vi "measconfig parse section.vi"(8 "error in (no error)":errorcluster, 10 "section name":string, 11 "refnum":T1) -> (0 "error out":errorcluster, 2 "measurement definition":T2={"sweep parameter"=enum."angle", "sweep start"=0.0, "sweep stop"=0.0, "sweep increment"=0.0, "temperature"=0.0, "path"=path "", "magnet initial"={"magnitude"=0.0, "phi"=0.0, "theta"=0.0}, "magnet reference"={"magnitude"=0.0, "phi"=0.0, "theta"=0.0}, "const phi?"=FALSE, "delta phi (deg)"=0.5, "delta H (mT)"=0.5, "const phi init field?"=FALSE}, 3 "refnum out":T1)   [LabVIEW 2013]
uses:
  <vilib>/Utility/config.llb/Config Data RefNum.ctl
  measconfig cluster.ctl
  measurement sweep parameter.ctl
  devices/magnet/magnet polar field.ctl
  <vilib>/Utility/config.llb/Read Key (String).vi
  <vilib>/Utility/config.llb/Read Key (Double).vi
  <vilib>/Utility/config.llb/NI_LVConfig.lvlib
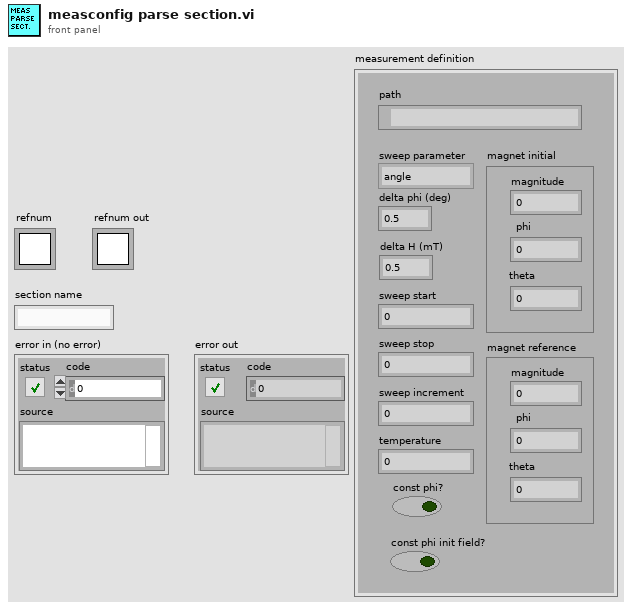
[diagram p1: front panel]
types:
  T1 = typedef "NI_LVConfig.lvlib/Config Data RefNum.ctl" = refnum<k1>
  T2 = typedef "measconfig cluster.ctl" = cluster{"sweep parameter":T3, "sweep start":dbl, "sweep stop":dbl, "sweep increment":dbl, "temperature":dbl, "path":path, "magnet initial":T4, "magnet reference":T4, "const phi?":bool, "delta phi (deg)":dbl, "delta H (mT)":dbl, "const phi init field?":bool}
  T3 = typedef "measurement sweep parameter.ctl" = enum16{"angle", "magnetic field"}
  T4 = typedef "magnet polar field.ctl" = cluster{"magnitude":dbl, "phi":dbl, "theta":dbl}
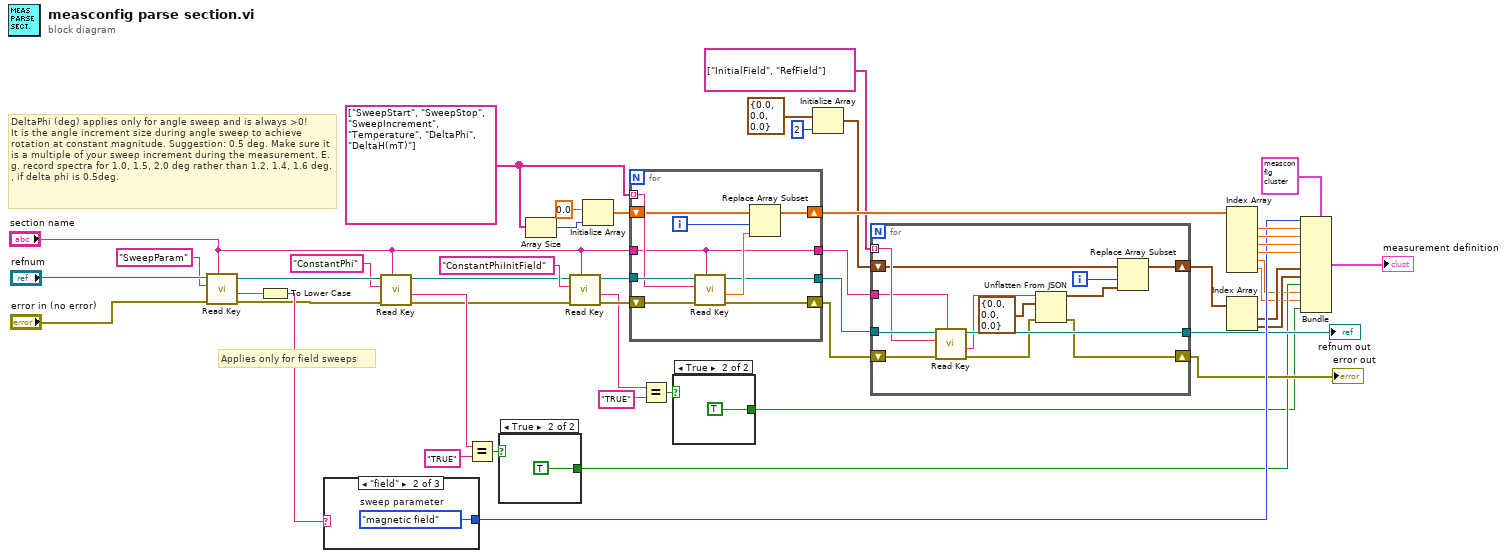
[diagram p0: block diagram]
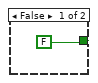
[diagram p2: hidden frame]
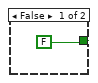
[diagram p3: hidden frame]
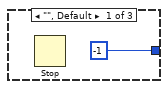
[diagram p4: hidden frame]
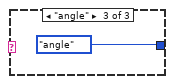
[diagram p5: hidden frame]
diagram:
  w34 = string[] ["SweepStart", "SweepStop", "SweepIncrement", "Temperature", "DeltaPhi", "DeltaH(mT)"]
  # "Applies only for field sweeps"
  # "DeltaPhi (deg) applies only for angle sweep and is always >0! \nIt is the angle increment size during angle sweep to achieve rotation at constant magnitude. Suggestion: 0.5 deg. Make sure it is a multiple of your sweep increment during the measurement. E.g. record spectra for 1.0, 1.5, 2.0 deg rather than 1.2, 1.4, 1.6 deg., if delta phi is 0.5deg."
  n1 = call-poly <vilib>:"Read Key.vi"("section"="section name", "error in (no error)"="error in (no error)", "key"="SweepParam", "refnum"="refnum") -> ("error out"=w19:errorcluster, "value"=w45:string, "refnum out"=w18:T1)  [unwired: 4 in, 1 out]
  n2 = To Lower Case(string=w45) -> (all lower case string=w44:string)
  n3 = case shown="\"field\"" w44 {
    tunnel: [-1 w50 enum16{"angle", "magnetic field", "temperature"}."angle" ("sweep parameter")] -> w36
    frame "", Default {
      n4 = Stop() -> ()  [unwired: 1 in]
    }
    frame "field" {
      w50 = measurement_sweep_parameter."magnetic field"  # sweep parameter
    }
    frame "angle" {
    }
  }
  n5 = call-poly <vilib>:"Read Key.vi"("section"="section name", "error in (no error)"=w19, "key"="ConstantPhi", "refnum"=w18) -> ("error out"=w8:errorcluster, "value"=w14:string, "refnum out"=w7:T1)  [unwired: 4 in, 1 out]
  n6 = Equal?(x=w14, y="TRUE") -> (x = y?=w15:bool)
  n7 = case shown="True" w15 {
    tunnel: [FALSE ("const phi?") TRUE ("const phi?")] -> w13
    frame False {
    }
    frame True {
    }
  }
  n8 = Array Size(array=w34) -> (size(s)=w33:i32)
  n9 = call-poly <vilib>:"Read Key.vi"("section"="section name", "error in (no error)"=w8, "key"="ConstantPhiInitField", "refnum"=w7) -> ("error out"=w9:errorcluster, "value"=w4:string, "refnum out"=w3:T1)  [unwired: 4 in, 1 out]
  n10 = Initialize Array(0.0, w33) -> (w42:dbl[])
  n11 = for {
    tunnel: w34 -> [w61] mode=indexing
    tunnel: w3 -> [w62]
    tunnel: "section name" -> [w54]
    shift-right: [w57] -> w41
    shift-left: w42 -> [w60]
    shift-right: [w56] -> w28
    shift-left: w9 -> [w63]
    tunnel: [w55] -> w29
    tunnel: [w54] -> w30
    i -> [w59]
    n12 = call-poly <vilib>:"Read Key.vi"("section"=w54, "error in (no error)"=w63, "key"=w61, "refnum"=w62) -> ("error out"=w56:errorcluster, "value"=w58:dbl, "refnum out"=w55:T1)  [unwired: 4 in, 1 out]
    n13 = Replace Array Subset(array=w60, new element=w58, index=w59) -> (w57:dbl[])
  }
  n14 = Equal?(x=w4, y="TRUE") -> (x = y?=w5:bool)
  n15 = case shown="True" w5 {
    tunnel: [FALSE ("const phi?") TRUE ("const phi?")] -> w2
    frame False {
    }
    frame True {
    }
  }
  n16 = Initialize Array(T4 {"magnitude"=0.0, "phi"=0.0, "theta"=0.0} ("magnet polar"), 2 ("dimension size")) -> (w20:T4[])
  n17 = for {
    tunnel: string[] ["InitialField", "RefField"] -> [w76] mode=indexing
    tunnel: w29 -> [w77]
    tunnel: w30 -> [w71]
    shift-right: [w73] -> w25
    shift-left: w20 -> [w75]
    shift-right: [w68] -> w26
    shift-left: w28 -> [w78]
    tunnel: [w72] -> w27
    i -> [w74]
    n18 = call-poly <vilib>:"Read Key.vi"("section"=w71, "error in (no error)"=w78, "key"=w76, "refnum"=w77) -> ("error out"=w69:errorcluster, "value"=w70:string, "refnum out"=w72:T1)  [unwired: 4 in, 1 out]
    n19 = Unflatten From JSON(JSON string=w70, type and defaults=T4 {"magnitude"=0.0, "phi"=0.0, "theta"=0.0} ("magnet polar"), error in (no error)=w69) -> (value=w66:T4, error out=w68:errorcluster)  [unwired: 4 in]
    n20 = Replace Array Subset(array=w75, new element=w66, index=w74) -> (w73:T4[])
  }
  "error out" <- w26
  "refnum out" <- w27
  n21 = Index Array(array=w41) -> (element #1=w40:dbl, element #2=w39:dbl, element #3=w38:dbl, element #4=w37:dbl, element #5=w12:dbl, element #6=w11:dbl)  [unwired: 6 in]
  n22 = Index Array(array=w25) -> (element #1=w24:T4, element #2=w23:T4)  [unwired: 2 in]
  n23 = Bundle(cluster=T2 {"sweep parameter"=enum."magnetic field", "sweep start"=0.1, "sweep stop"=1.0, "sweep increment"=0.1, "temperature"=0.0, "path"=path "", "magnet initial"={"magnitude"=0.0, "phi"=0.0, "theta"=0.0}, "magnet reference"={"magnitude"=0.0, "phi"=0.0, "theta"=0.0}, "const phi?"=FALSE, "delta phi (deg)"=0.0, "delta H (mT)"=0.0, "const phi init field?"=FALSE} ("measurement definition"), "sweep parameter"=w36, "sweep start"=w40, "sweep stop"=w39, "sweep increment"=w38, "temperature"=w37, "magnet initial"=w24, "magnet reference"=w23, "const phi?"=w13, "delta phi (deg)"=w12, "delta H (mT)"=w11, "const phi init field?"=w2) -> (→"measurement definition":T2)  [unwired: 1 in]
